vi "Do Request.vi"(7 "Processing In":refnum<class "Processing.lvclass">, 11 "Challenges in":refnum<class "Challenges.lvclass">) -> (0 "error out":errorcluster, 5 "Processing":refnum<class "Processing.lvclass">)   [LabVIEW 2020, in "Summer of LabVIEW.lvlib" / "Challenges.lvclass"]
uses:
  Challenges.lvclass
  <vilib>/IlluminatedG/IG HTTP Server/HTTP Server/Processing/Processing.lvclass
  Challenge DB/Challenge DB.lvclass
  <vilib>/IlluminatedG/IG HTTP Server/HTTP Server/Security/Security.lvclass
  <vilib>/IlluminatedG/IG HTTP Server/HTTP Server/Processing/Processing.lvclass/Processing.ctl
  Data Types/Challenge JSON.ctl
  dc6fd1d0-de9f-4401-8f8b-b5c32b4ea38c.vi
  2f66f478-f322-4db6-a85b-38a2410aa250.vi
  8988f826-3dc3-4306-b390-a1ad4cd6b336.vi
  dc6fd1d0-de9f-4401-8f8b-b5c32b4ea38c.vi/9528e9df-aefc-4ce0-9221-106a337fd3b6.vi
  2f66f478-f322-4db6-a85b-38a2410aa250.vi/36b1f833-cfc6-44a5-864d-b53e3b32e5c8.vi
  8988f826-3dc3-4306-b390-a1ad4cd6b336.vi/9528e9df-aefc-4ce0-9221-106a337fd3b6.vi
  <vilib>/IlluminatedG/IG HTTP Server/HTTP Server/Values/Get Arg Map.vi
  <vilib>/Utility/error.llb/Error Cluster From Error Code.vi
  Challenge/Challenge.lvclass
  Challenges.lvclass/Challenges.ctl
  Summer of LabVIEW.lvlib
  <vilib>/IlluminatedG/IG HTTP Utils/HTTP Utils/Response/Response.lvclass
  <vilib>/IlluminatedG/lv-web-crypto/lv-json/JSON/JSON.lvlib
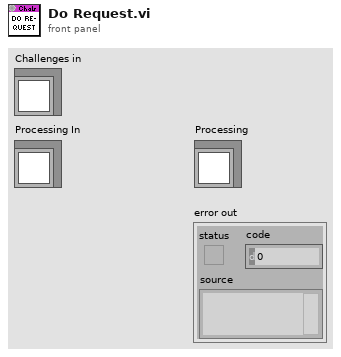
[diagram p1: front panel]
types:
  T1 = typedef "Summer of LabVIEW.lvlib/Challenge JSON.ctl" = cluster{"id":i64, "name":string, "description":string, "download":string, "instructions":string, "start":string, "end":string}
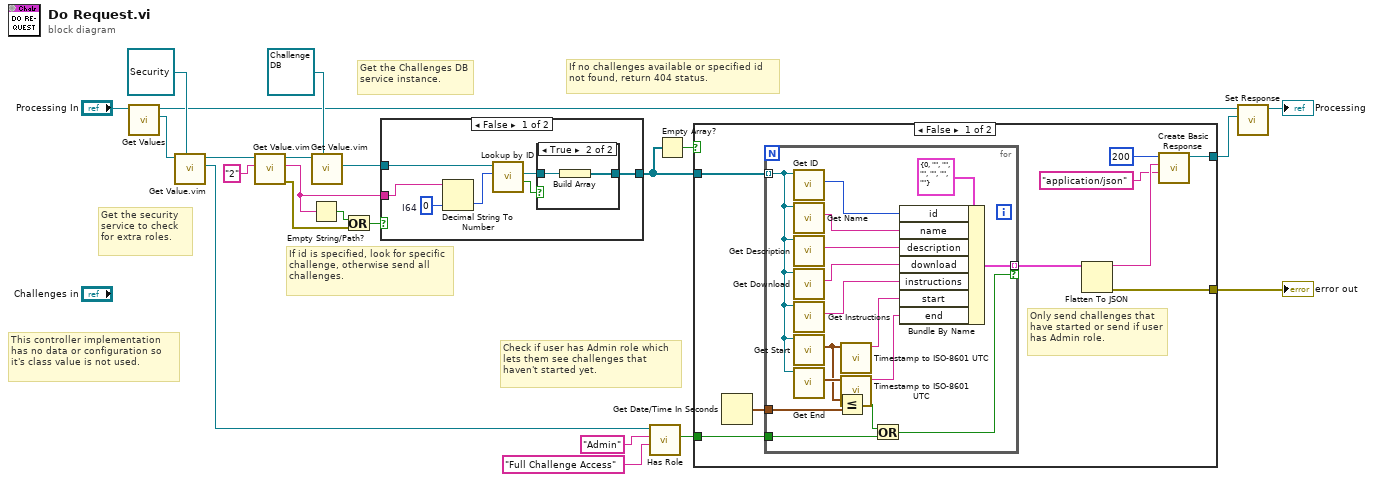
[diagram p0: block diagram]
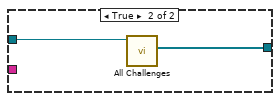
[diagram p3: hidden frame]
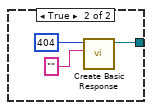
[diagram p4: hidden frame]
diagram:
  # "If no challenges available or specified id not found, return 404 status."
  # "This controller implementation has no data or configuration so it's class value is not used."
  # "Get the security service to check for extra roles."
  # "Get the Challenges DB service instance."
  # "Check if user has Admin role which lets them see challenges that haven't started yet."
  # "If id is specified, look for specific challenge, otherwise send all challenges."
  n1 = call <vilib>:"Get Values.vi"("Processing in"="Processing In") -> ("Values"=w18:refnum<class "Values.lvclass">, "Processing out"=w8:refnum<class "Processing.lvclass">)  [unwired: 9 in]
  n2 = call "Get Value.vim"("Type / Server / Service (String)"=refnum<class "Security.lvclass"> refnum ("HTTP Server.lvlib:Security.lvclass"), "Arguments in"=w18) -> ("Value"=w16:refnum<class "Security.lvclass">, "Arguments out"=w7:refnum<class "Values.lvclass">)  [unwired: 7 in, 1 out]
  n3 = call "Get Value.vim"("Name for Type"="2", "Arguments in"=w7) -> ("error out"=w2:errorcluster, "Value"=w4:string, "Arguments out"=w5:refnum<class "Values.lvclass">)  [unwired: 7 in]
  n4 = Empty String/Path?(string/path=w4) -> (empty?=w3:bool)
  n5 = call "Get Value.vim"("Type / Server / Service (String)"=refnum<class "Challenge DB.lvclass"> refnum ("SOL:Challenge DB.lvclass"), "Arguments in"=w5) -> ("Value"=w20:refnum<class "Challenge DB.lvclass">)  [unwired: 7 in, 2 out]
  n6 = Or(x=w3, y=w2) -> (x .or. y?=w1:bool)
  n7 = case shown="False" w1 {
    tunnel: w20 -> [w29 w33]
    tunnel: [w26 w32] -> w11
    tunnel: w4 -> [w25 _]
    frame False {
      w24 = i64 0  # I64
      n8 = Decimal String To Number(string=w25, default (0L)=w24) -> (number=w23:i64)  [unwired: 1 in, 1 out]
      n9 = call "Lookup by ID.vi"("ID"=w23, "Challenge DB in"=w29) -> ("Found?"=w28:bool, "Challenge"=w27:refnum<class "Challenge.lvclass">)  [unwired: 6 in, 2 out]
      n10 = case shown="True" w28 {
        tunnel: w27 -> [_ w31]
        tunnel: [_ w30] -> w26
        frame False {
        }
        frame True {
          n11 = Build Array(w31) -> (w30:refnum<class "Challenge.lvclass">[])
        }
      }
    }
    frame True {
      n12 = call "All Challenges.vi"("Challenge DB in"=w33) -> ("Challenges"=w32:refnum<class "Challenge.lvclass">[])  [unwired: 8 in, 2 out]
    }
  }
  n13 = call <vilib>:"Has Role.vi"("Description (None)"="Full Challenge Access" ("Role"), "Role"="Admin", "Security in"=w16) -> ("Has Role?"=w9:bool)  [unwired: 6 in, 2 out]
  n14 = Empty Array?(array=w11) -> (empty?=w10:bool)
  n15 = case shown="False" w10 {
    tunnel: [w39 w61] -> w13
    tunnel: [w38 _] -> w12
    tunnel: w9 -> [w36 _]
    tunnel: w11 -> [w34 _]
    frame False {
      # "Only send challenges that have started or send if user has Admin role."
      n16 = Get Date/Time In Seconds() -> (seconds since 1Jan1904=w35:timestamp)
      n17 = for {
        tunnel: w34 -> [w51] mode=indexing
        tunnel: [w52] -> w37 mode=indexing if=w45
        tunnel: w36 -> [w44]
        tunnel: w35 -> [w43]
        n18 = call "Get ID.vi"("Challenge in"=w51) -> ("ID"=w55:i64)  [unwired: 9 in, 1 out]
        n19 = call "Get Name.vi"("Challenge in"=w51) -> ("Name"=w56:string)  [unwired: 9 in, 1 out]
        n20 = call "Get Description.vi"("Challenge in"=w51) -> ("Description"=w57:string)  [unwired: 9 in, 1 out]
        n21 = call "Get Download.vi"("Challenge in"=w51) -> ("Download"=w54:string)  [unwired: 9 in, 1 out]
        n22 = call "Get Instructions.vi"("Challenge in"=w51) -> ("Instructions"=w53:string)  [unwired: 9 in, 1 out]
        n23 = call "Get Start.vi"("Challenge in"=w51) -> ("Start"=w47:timestamp)  [unwired: 9 in, 1 out]
        n24 = call "Get End.vi"("Challenge in"=w51) -> ("End"=w50:timestamp)  [unwired: 9 in, 1 out]
        n25 = Less Or Equal?(x=w47, y=w43) -> (x <= y?=w46:bool)
        n26 = call <vilib>:"Timestamp to ISO-8601 UTC.vi"("Time Stamp"=w47) -> ("ISO 8601 UTC"=w49:string)  [unwired: 10 in]
        n27 = call <vilib>:"Timestamp to ISO-8601 UTC.vi"("Time Stamp"=w50) -> ("ISO 8601 UTC"=w48:string)  [unwired: 10 in]
        n28 = Or(x=w46, y=w44) -> (x .or. y?=w45:bool)
        n29 = Bundle By Name(cluster=T1 {"id"=0, "name"="", "description"="", "download"="", "instructions"="", "start"="", "end"=""} ("Challenge JSON"), "id"=w55, "name"=w56, "description"=w57, "download"=w54, "instructions"=w53, "start"=w49, "end"=w48) -> (w52:T1)
      }
      n30 = Flatten To JSON(anything=w37) -> (JSON string=w42:string, 11:w38:errorcluster)  [unwired: 2 in]
      n31 = call <vilib>:"Create Basic Response.vi"("Content-Type (text/plain)"="application/json", "Payload"=w42, "Status Code"=u16 200) -> ("Response out"=w39:refnum<class "Response.lvclass">)  [unwired: 7 in, 1 out]
    }
    frame True {
      n32 = call <vilib>:"Create Basic Response.vi"("Payload"="", "Status Code"=u16 404) -> ("Response out"=w61:refnum<class "Response.lvclass">)  [unwired: 8 in, 1 out]
    }
  }
  "error out" <- w12
  n33 = call <vilib>:"Set Response.vi"("Response"=w13, "Processing in"=w8) -> ("Processing out"=→"Processing":refnum<class "Processing.lvclass">)  [unwired: 9 in]
